vi "XIPIN_ZYNQ7_Processing_System_5_5.vi"   [LabVIEW 2017]
doc: "Arm dual core SOC with Zynq fpga\n------------------------------------\n<b>Need License</b> : No\n<b>Interface</b> : AXI4 AXI4-Stream"
uses:
  <vilib>/rvi/XilinxIP/XIPIN_XNode/niFpgaXIPIN.xnode
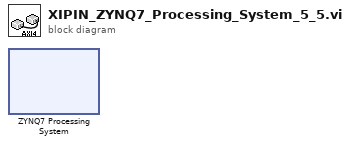
[diagram p0: block diagram]
diagram:
  n1 = xnode ("ZYNQ7 Processing System")() -> ()
